vi "1D experiment wii.vi"() -> ()   [LabVIEW 2011]
uses:
  <vilib>/Platform/TimedLoop/XDataNode/timing_clust.ctl
  <vilib>/Platform/TimedLoop/XDataNode/nitl_modes.ctl
  <vilib>/Platform/TimedLoop/XDataNode/wakeup.ctl
  3D_Experiment/libs/experiments 2/Action Engines/AE Access VIs/AE - Bluetooth Initialise.vi
  3D_Experiment/libs/experiments 2/Action Engines/AE Access VIs/AE - Bluetooth Connect All.vi
  <vilib>/Utility/inputDevices.llb/closeMouse.vi
  <vilib>/Utility/cursorutil.llb/Set Cursor (Cursor ID).vi
  <vilib>/Utility/inputDevices.llb/mouseAcquire.vi
  <vilib>/Utility/file.llb/Write To Spreadsheet File (DBL).vi
  <vilib>/Utility/file.llb/Write To Spreadsheet File (I64).vi
  <vilib>/Platform/TimedLoop/XDataNode/XDataNode.xnode
  <vilib>/Platform/TimedLoop/XDataNode/XDNodeRunTimeDep.lvlib
  User32.dll
panel:
  out "initial time":u32
  out "1D Experiment":cluster{"Y":dbl[], "Y":dbl[]}[](graph)
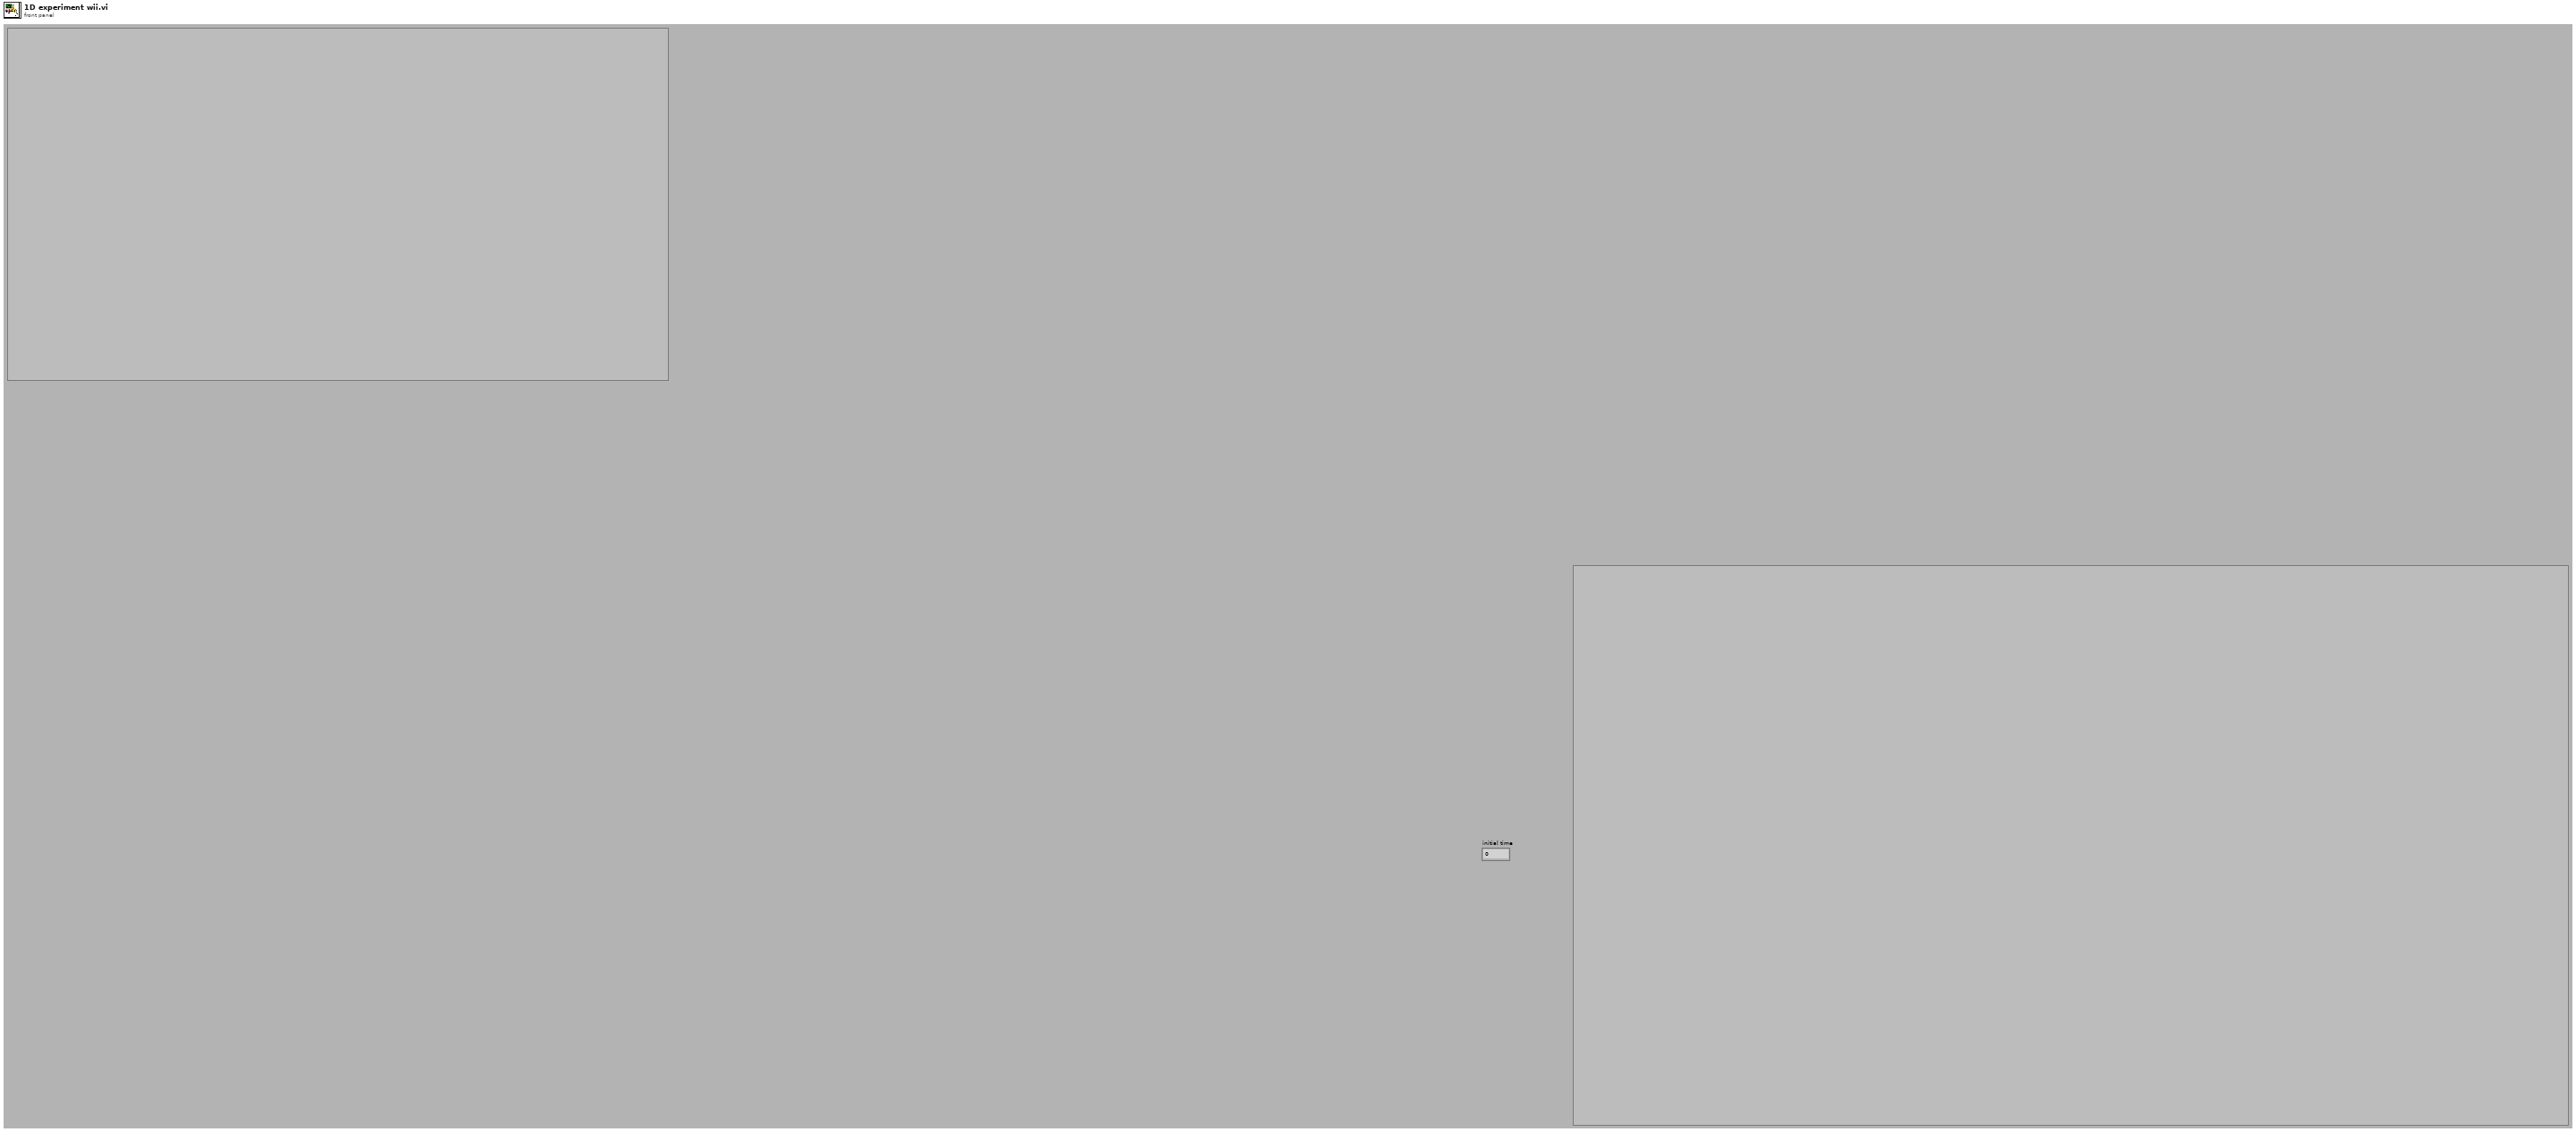
[diagram p1: front panel]
types:
  T1 = enum16{"open", "replace", "create", "open or create", "replace or create", "replace or create with confirmation"}
  T2 = typedef "XDNodeRunTimeDep.lvlib/timing_clust.ctl" = cluster{"Expected End [f-1]":u64, "Actual End [f-1]":u64, "Finished Late? [f-1]":bool, "Expected End [i-1]":u64, "Actual End [i-1]":u64, "Finished Late? [i-1]":bool, "Expected Start [i]":u64, "Actual Start [i]":u64, "Expected Start [f]":u64, "Actual Start [f]":u64, "Source Name":string, "Structure Name":string, "Period":i64, "Deadline":i64, "Offset":i64, "Start":i64, "Priority":i32, "Timeout":i32, "Mode":T3, "Wakeup Reason":T4, "Error":errorcluster, "Source Type":string, "Secondary Source Type":string, "Global End Time":u64, "Global Start Time":u64, "Frame Duration":u64, "Iteration Duration":u64, "Assigned CPU":i32, "I/O Scan Engine Mode":u32}
  T3 = typedef "XDNodeRunTimeDep.lvlib/nitl_modes.ctl" = enum32{"No Change", "Process missed periods, maintain original phase", "Discard missed periods, maintain original phase", "Process missed periods, ignore original phase", "Discard missed periods, ignore original phase"}
  T4 = typedef "XDNodeRunTimeDep.lvlib/wakeup.ctl" = enum32{"Normal", "Aborted", "Asynchronous wakeup", "Timing source error", "Timed loop error", "Timeout"}
  T5 = cluster{"Radius":dbl, "x0":dbl, "y0":dbl, "D":dbl, bool}
  T6 = typedef "LVAllMonitorsDisplayTypeDef.ctl" = cluster{"Bounds":cluster{"Left":i16, "Top":i16, "Right":i16, "Bottom":i16}, "Depth":i16}[]
  T7 = cluster{"Bounds":cluster{"Left":i16, "Top":i16, "Right":i16, "Bottom":i16}, "Depth":i16}
  T8 = cluster{"Left":i16, "Top":i16, "Right":i16, "Bottom":i16}
  T9 = cluster{"Horizontal":i32, "Vertical":i32, "Scrolling":i32}
  T10 = cluster{"button 1":bool, "button 2":bool, "button 3":bool, "button 4":bool}
  T11 = typedef "LVPoint32TypeDef.ctl" = cluster{"Horizontal":i32, "Vertical":i32}
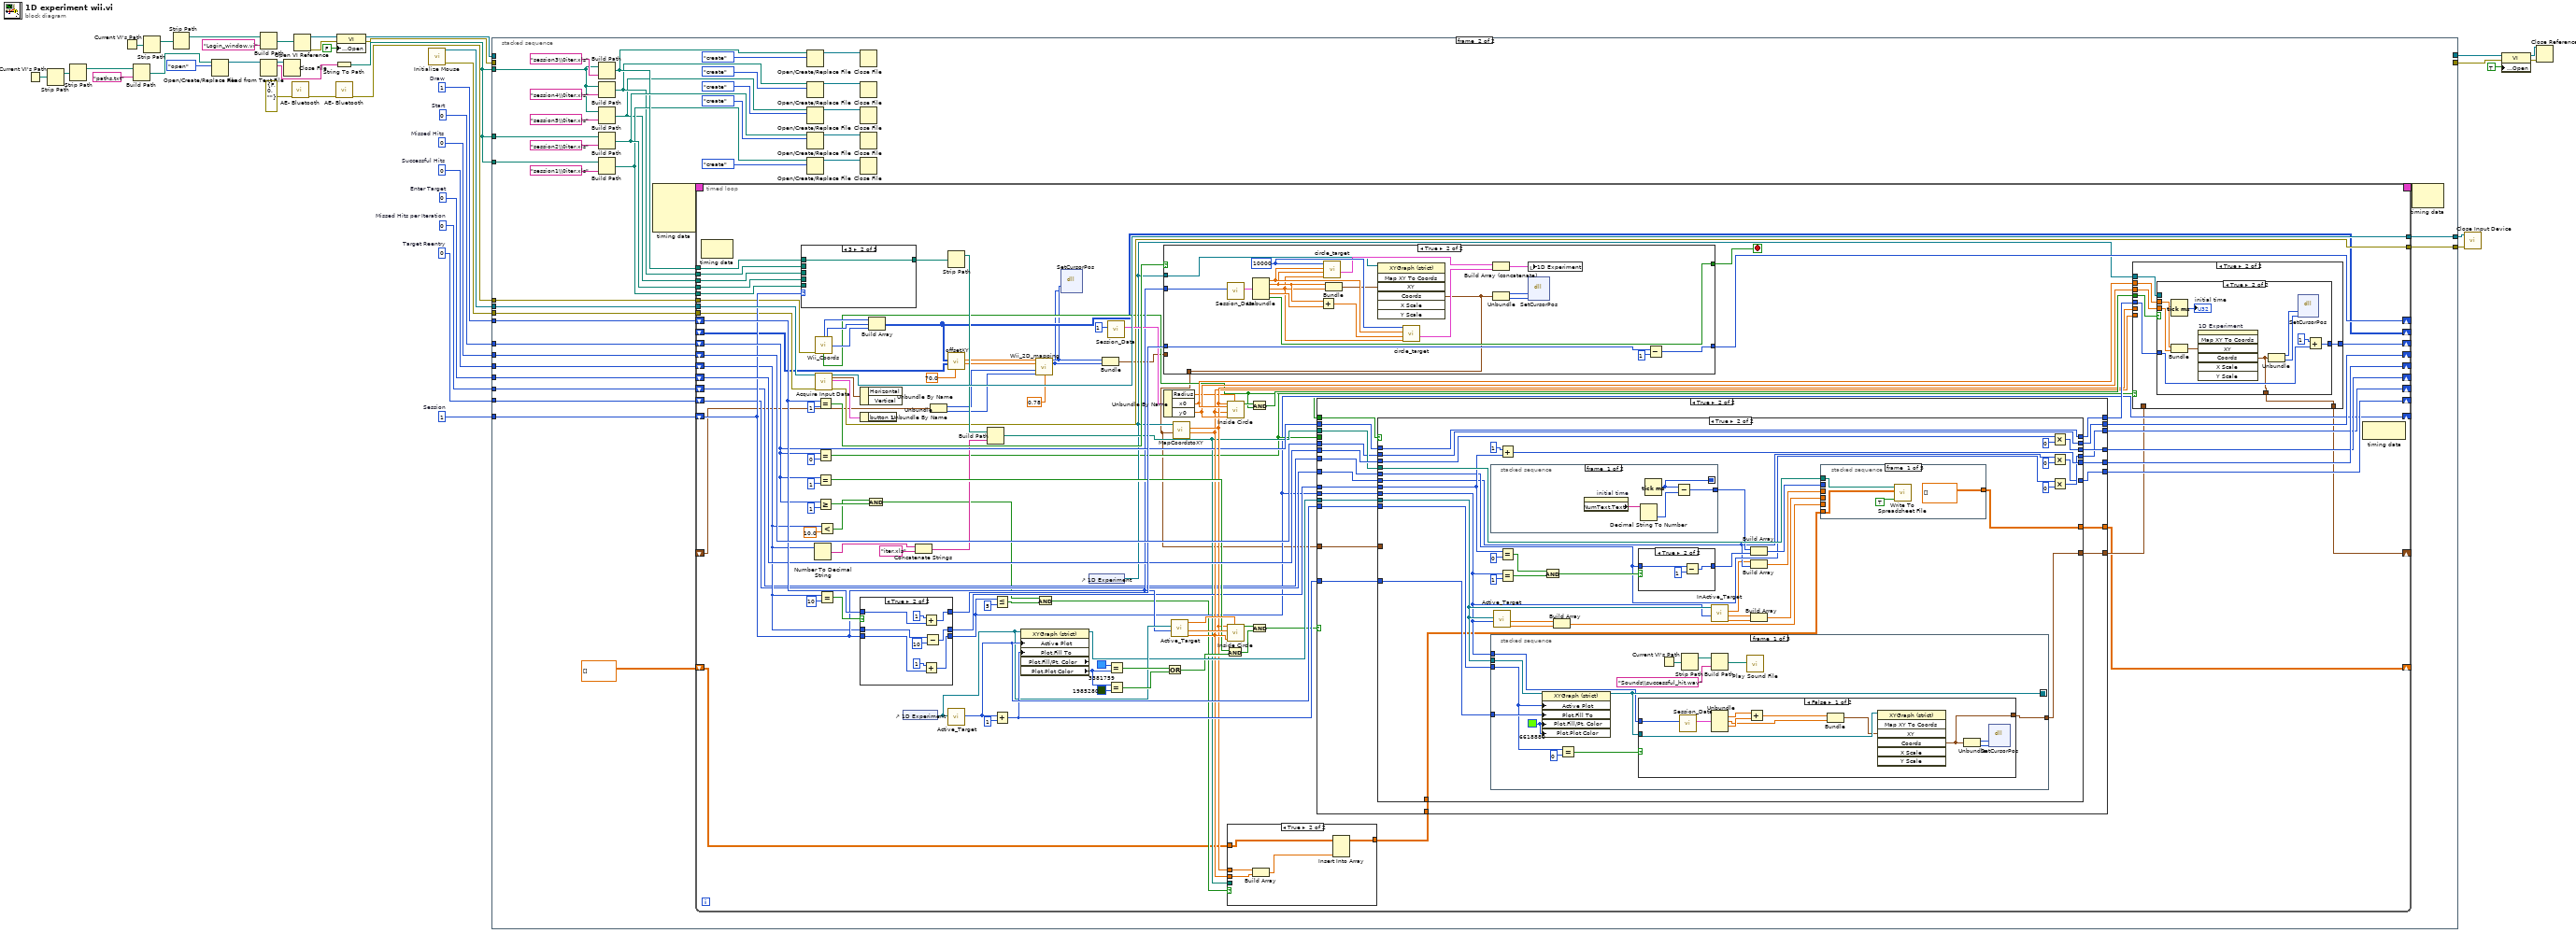
[diagram p0: block diagram]
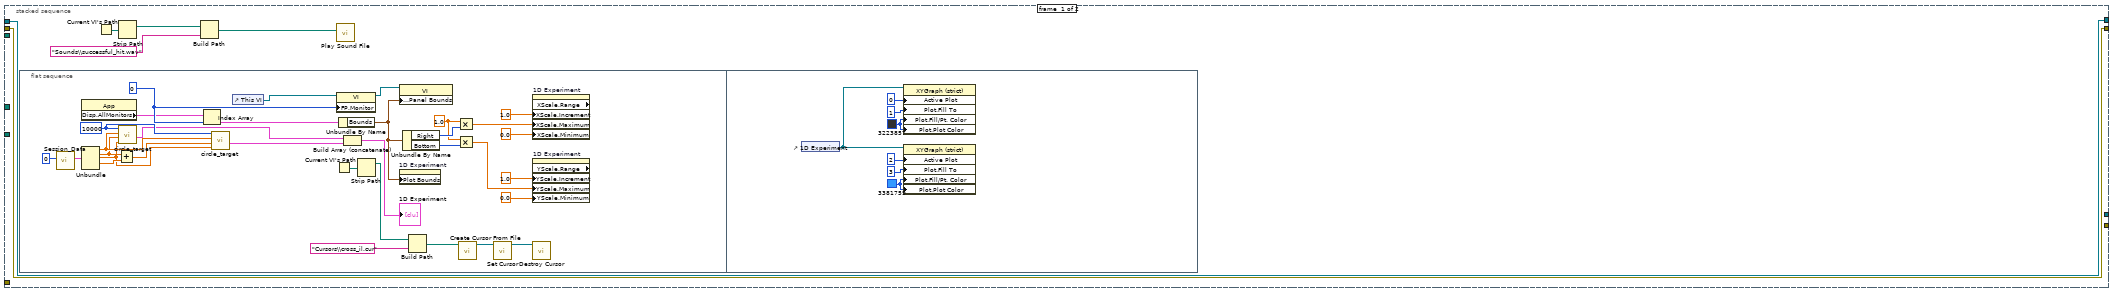
[diagram p2: hidden frame]
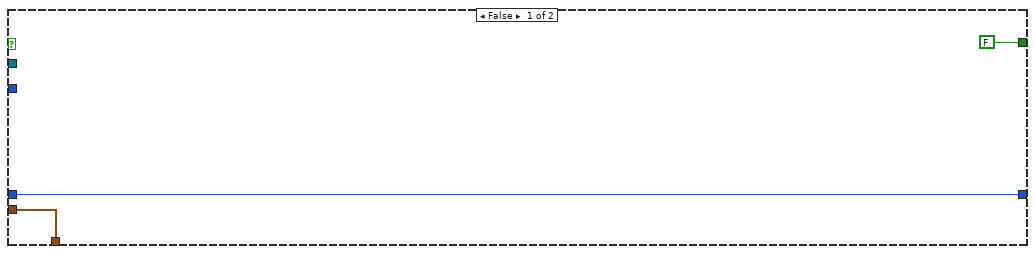
[diagram p8: hidden frame]
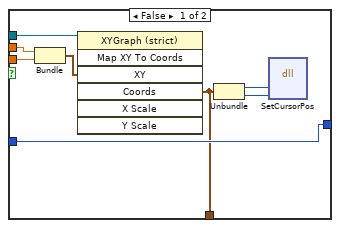
[diagram p10: hidden frame]
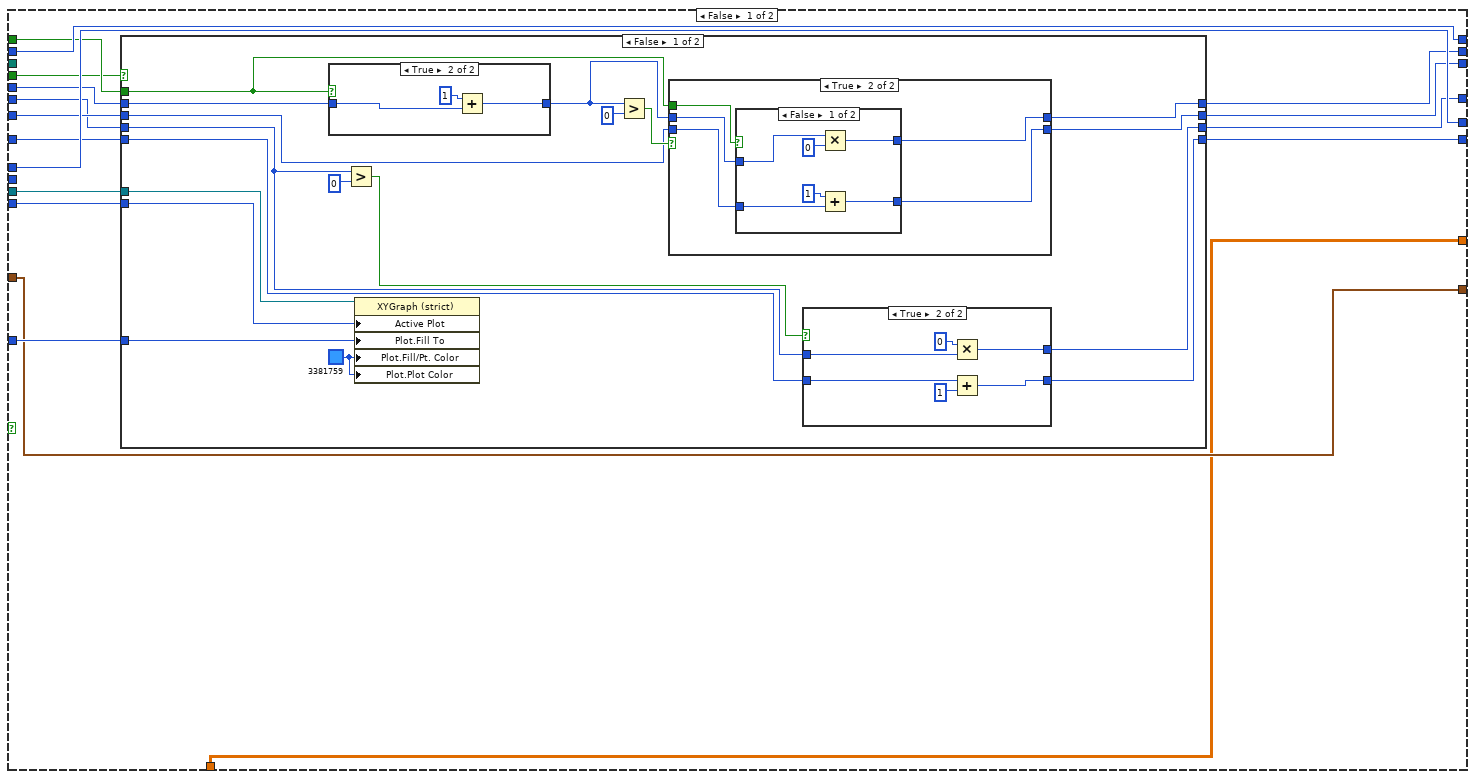
[diagram p12: hidden frame]
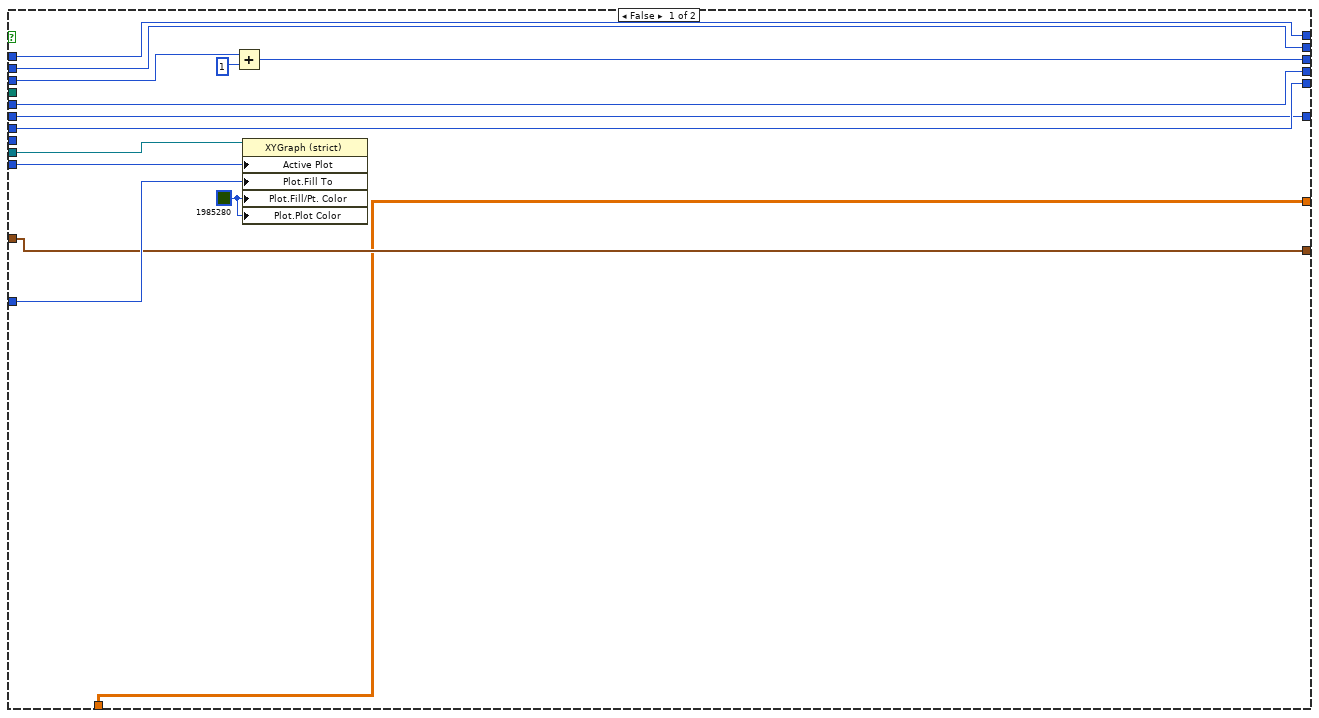
[diagram p18: hidden frame]
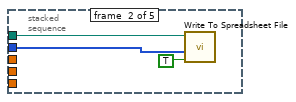
[diagram p20: hidden frame]
diagram:
  w6 = 0  # Target Reentry
  w7 = 0  # Missed Hits per Iteration
  w33 = 0  # Enter Target
  w34 = 1  # Draw
  w35 = 0  # Start
  w36 = 1  # Session
  w37 = 0  # Missed Hits
  w38 = 0  # Successful Hits
  n1 = Current VI's Path() -> (path=w15:path)
  n2 = Strip Path(path=w15) -> (stripped path=w10:path)  [unwired: 1 out]
  n3 = Strip Path(path=w10) -> (stripped path=w11:path)  [unwired: 1 out]
  n4 = Current VI's Path() -> (path=w18:path)
  n5 = Build Path(base path=w11, name or relative path="paths.txt") -> (appended path=w13:path)
  n6 = Strip Path(path=w18) -> (stripped path=w8:path)  [unwired: 1 out]
  n7 = Strip Path(path=w8) -> (stripped path=w9:path)  [unwired: 1 out]
  n8 = Open/Create/Replace File(file path (use dialog)=w13, operation (0:open)=T1."open") -> (refnum out=w31:refnum<file>)  [unwired: 4 in, 2 out]
  n9 = Build Path(base path=w9, name or relative path="Login_window.vi") -> (appended path=w16:path)
  n10 = Read from Text File(file (use dialog)=w31) -> (refnum out=w32:refnum<file>, text=w30:string)  [unwired: 3 in, 2 out]
  n11 = Close File(refnum=w32) -> ()  [unwired: 1 in, 2 out]
  n12 = call-poly "AE- Bluetooth.vi"("error in (no error)"=errorcluster {"status"=FALSE, "code"=0, "source"=""}) -> ("error out"=w2:errorcluster)  [unwired: 10 in]
  n13 = Open VI Reference(vi path=w16) -> (vi reference=w28:refnum<vi>, error out=w27:errorcluster)  [unwired: 5 in]
  n14 = String To Path(string=w30) -> (path=w29:path)
  n15 = call-poly "AE- Bluetooth.vi"("error in (no error)"=w2) -> ("error out"=w1:errorcluster)  [unwired: 9 in, 1 out]
  n16 = property class="VI"(reference=w28, error in=w27, "Front Panel Window:Open"=FALSE) -> (reference out=w25:refnum<vi>, error out=w24:errorcluster)
  n17 = call <vilib>:"Initialize Mouse.vi"() -> ("error out"=w5:errorcluster, "device ID"=w40:refnum<k1>)  [unwired: 1 in, 9 out]
  n18 = stacked-sequence {
    tunnel: w40 -> [_ w124]
    tunnel: [_ w123] -> w39
    tunnel: w38 -> [_ w122]
    tunnel: w37 -> [_ w121]
    tunnel: w36 -> [_ w117]
    tunnel: w35 -> [_ w120]
    tunnel: w34 -> [_ w119]
    tunnel: w33 -> [_ w118]
    tunnel: w29 -> [_ w107]
    tunnel: w29 -> [_ w114]
    tunnel: w29 -> [_ w94]
    tunnel: w25 -> [w42 _]
    tunnel: w24 -> [w41 _]
    tunnel: [w42 _] -> w20
    tunnel: [w41 _] -> w19
    tunnel: w7 -> [_ w100]
    tunnel: w6 -> [_ w99]
    tunnel: w5 -> [_ w98]
    tunnel: [_ w97] -> w4
    tunnel: w1 -> [_ w87]
    frame #0 {
      n19 = flat-sequence {
        frame #0 {
          w64 = 1.0 ("y")
          w69 = u16 0 ("Front Panel Window:Monitor")
          w78 = 10000
          n20 = call "Session_Data.vi"("Session"=0) -> ("output cluster"=w56:T5)  [unwired: 10 in]
          n21 = property class="App"() -> ("Disp.AllMonitors"=w68:T6)  [unwired: 2 in, 2 out]
          n22 = Unbundle(w56) -> ("Radius"=w76:dbl, "x0"=w54:dbl, "y0"=w53:dbl, "D"=w55:dbl)  [unwired: 1 out]
          n23 = Add(x=w54, y=w55) -> (x+y=w77:dbl)
          n24 = call "circle_target.vi"("y0"=w53, "x0"=w54, "Radius"=w76, "Pixels"=w78) -> ("Target plots"=w74:cluster{dbl[], dbl[]}[])  [unwired: 7 in]
          n25 = Index Array(array=w68, index=w69) -> (element=w70:T7)
          n26 = call "circle_target.vi"("y0"=w53, "x0"=w77, "Radius"=w76, "Pixels"=w78) -> ("Target plots"=w75:cluster{dbl[], dbl[]}[])  [unwired: 7 in]
          n27 = control-ref of="This VI"() -> (w71:refnum<vi>)
          n28 = Current VI's Path() -> (path=w52:path)
          n29 = property class="VI"(reference=w71, "FP.Monitor"=w69) -> (reference out=w67:refnum<vi>)  [unwired: 1 in, 1 out]
          n30 = Unbundle By Name(w70) -> ("Bounds"=w66:T8)
          n31 = Build Array (concatenate)(w74, w75) -> (→"1D Experiment":cluster{dbl[], dbl[]}[])
          n32 = Strip Path(path=w52) -> (stripped path=w51:path)  [unwired: 1 out]
          n33 = property class="VI"(reference=w67, "Front Panel Window:Panel Bounds"=w66) -> ()  [unwired: 1 in, 2 out]
          n34 = property on="1D Experiment" class="XYGraph (strict)"("Plot Bounds"=w66) -> ()  [unwired: 2 in, 2 out]
          n35 = Unbundle By Name(w66) -> ("Right"=w65:i16, "Bottom"=w63:i16)
          n36 = Build Path(base path=w51, name or relative path="Cursors\\cross_il.cur") -> (appended path=w49:path)
          n37 = Multiply(x=w64, y=w65) -> (x*y=w61:dbl)
          n38 = Multiply(x=w64, y=w63) -> (x*y=w58:dbl)
          n39 = call <vilib>:"Create Cursor From File.vi"("cursor file"=w49) -> ("cursor ID"=w48:refnum<k1>)  [unwired: 9 in, 1 out]
          n40 = call-poly <vilib>:"Set Cursor.vi"("cursor ID"=w48) -> ("previous cursor ID"=w47:refnum<k1>)  [unwired: 9 in, 1 out]
          n41 = property on="1D Experiment" class="XYGraph (strict)" props=["XScale", "Range", "XScale", "Increment", "XScale", "Maximum", "XScale", "Minimum"]("XScale.Increment"=1.0 ("X Scale.Range:Increment"), "XScale.Maximum"=w61, "XScale.Minimum"=0.0 ("X Scale.Range:Minimum")) -> ()  [unwired: 2 in, 3 out]
          n42 = property on="1D Experiment" class="XYGraph (strict)" props=["YScale", "Range", "YScale", "Increment", "YScale", "Maximum", "YScale", "Minimum"]("YScale.Increment"=1.0 ("Y Scale.Range:Increment"), "YScale.Maximum"=w58, "YScale.Minimum"=0.0 ("Y Scale.Range:Minimum")) -> ()  [unwired: 2 in, 3 out]
          n43 = call <vilib>:"Destroy Cursor.vi"("cursor ID"=w47) -> ()  [unwired: 9 in, 1 out]
        }
        frame #1 {
          w84 = u32 3381759
          w81 = u32 3223857
          n44 = control-ref of="1D Experiment"() -> (w85:refnum<vi>)
          n45 = property on="Property Node" class="XYGraph (strict)"(reference=w85, "Active Plot"=u32 0, "Plot.Fill To"=i16 1, "Plot.Fill/Pt. Color"=w81, "Plot.Plot Color"=w81) -> ()  [unwired: 1 in, 2 out]
          n46 = property on="Property Node" class="XYGraph (strict)"(reference=w85, "Active Plot"=u32 2, "Plot.Fill To"=i16 3, "Plot.Fill/Pt. Color"=w84, "Plot.Plot Color"=w84) -> ()  [unwired: 1 in, 2 out]
        }
      }
      n47 = Current VI's Path() -> (path=w44:path)
      n48 = Strip Path(path=w44) -> (stripped path=w43:path)  [unwired: 1 out]
      n49 = Build Path(base path=w43, name or relative path="Sounds\\successful_hit.wav") -> (appended path=w45:path)
      n50 = call <vilib>:"Play Sound File.vi"("path"=w45) -> ()  [unwired: 9 in, 2 out]
    }
    frame #1 {
      n51 = Build Path(base path=w94, name or relative path="session3\\0iter.xls") -> (appended path=w108:path)
      n52 = Build Path(base path=w94, name or relative path="session4\\0iter.xls") -> (appended path=w89:path)
      n53 = Build Path(base path=w94, name or relative path="session5\\0iter.xls") -> (appended path=w88:path)
      n54 = Build Path(base path=w114, name or relative path="session2\\0iter.xls") -> (appended path=w111:path)
      n55 = Build Path(base path=w107, name or relative path="session1\\0iter.xls") -> (appended path=w103:path)
      n56 = node-c288() -> (w102:T2)  [unwired: 4 in]
      n57 = timed-loop {
        tunnel: w124 -> [w217]
        tunnel: [w216] -> w123
        shift-right: [w214] -> _
        shift-left: w122 -> [w165]
        shift-right: [w212] -> _
        shift-left: w121 -> [w213]
        shift-right: [w156] -> _
        shift-left: w117 -> [w178]
        shift-right: [w204] -> _
        shift-left: w120 -> [w181]
        shift-right: [w198] -> _
        shift-left: w119 -> [w199]
        shift-right: [w194] -> _
        shift-left: w118 -> [w195]
        tunnel: w103 -> [w179]
        tunnel: w111 -> [w177]
        tunnel: w108 -> [w176]
        timing: w102 -> [_]
        timing-out: [_] -> w101
        shift-right: [w161] -> _
        shift-left: w100 -> [w163]
        shift-right: [w159] -> _
        shift-left: w99 -> [w160]
        tunnel: w98 -> [w151]
        tunnel: [w150] -> w97
        tunnel: w89 -> [w149]
        tunnel: w88 -> [w148]
        tunnel: w87 -> [w143]
        shift-right: [w139] -> _
        shift-left: _ -> [w138]
        shift-right: [w130] -> _
        shift-left: _ -> [w134]
        shift-right: [w125] -> _
        shift-left: dbl[][] [] -> [w127]
        stop <- w188 stop-if-true
        n58 = node-c288() -> ()  [unwired: 1 in, 1 out]
        n59 = case shown="3" w178 {
          tunnel: w179 -> [_ _ _ _ w234]
          tunnel: [w230 w231 w232 w233 w234] -> w174
          tunnel: w177 -> [w230 _ _ _ _]
          tunnel: w176 -> [_ w231 _ _ _]
          tunnel: w149 -> [_ _ w232 _ _]
          tunnel: w148 -> [_ _ _ w233 _]
          frame 2 {
          }
          frame 3 {
          }
          frame 4 {
          }
          frame 5 {
          }
          frame 1, Default {
          }
        }
        n60 = Number To Decimal String(number=w165) -> (decimal integer string=w173:string)  [unwired: 1 in]
        n61 = call "Wii_Coords.vi"("error in (no error)"=w143) -> ("Raw X Values"=w147:i32[], "Raw Y Values"=w146:i32[], "Sizes"=w145:i32[], "B"=w142:bool)  [unwired: 7 in, 4 out]
        n62 = call-poly <vilib>:"Acquire Input Data.vi"("device ID"=w217, "error in (no error)"=w151) -> ("device ID"=w216:refnum<k1>, "axis info"=w215:T9, "button info"=w218:T10, "error out"=w150:errorcluster)  [unwired: 1 in, 13 out]
        n63 = Equal?(x=w199, y=1) -> (x = y?=w196:bool)
        n64 = Equal?(x=w181, y=0) -> (x = y?=w162:bool)
        n65 = Equal?(x=w181, y=1) -> (x = y?=w190:bool)
        n66 = Greater Or Equal?(x=w181, y=1) -> (x >= y?=w168:bool)
        n67 = Less?(x=w165, y=10.0) -> (x < y?=w167:bool)
        n68 = Equal?(x=w165, y=10) -> (x = y?=w210:bool)
        n69 = Unbundle By Name(w215) -> ()  [unwired: 2 out]
        n70 = Unbundle By Name(w218) -> ()  [unwired: 1 out]
        n71 = case shown="True" w210 {
          tunnel: w165 -> [w293 w302]
          tunnel: [w293 w300] -> w175
          tunnel: w178 -> [w292 w294]
          tunnel: [w292 w295] -> w156
          tunnel: w199 -> [w291 w298]
          tunnel: [w291 w296] -> w197
          frame False {
          }
          frame True {
            n72 = Add(x=1, y=w298) -> (x+y=w296:i32)
            n73 = Add(x=1, y=w294) -> (x+y=w295:i32)
            n74 = Subtract(x=w302, y=10) -> (x-y=w300:i32)
          }
        }
        n75 = And(x=w167, y=w168) -> (x .and. y?=w157:bool)
        n76 = Build Array(w147, w146, w145) -> (w139:i32[][])
        n77 = control-ref of="1D Experiment"() -> (w208:refnum<vi>)
        n78 = Concatenate Strings(w173, "iter.xls" ("name or relative path")) -> (w171:string)
        n79 = Unbundle(w134) -> ("Horizontal"=w133:i32, "Vertical"=w132:i32)
        n80 = Strip Path(path=w174) -> (stripped path=w170:path)  [unwired: 1 out]
        n81 = call "offsetXY.vi"("Thres"=70.0, "Previous"=w138, "Current"=w139) -> ("OffsetY"=w141:dbl, "OffsetX"=w140:dbl)  [unwired: 7 in]
        n82 = call "Active_Target.vi"("XYGraph Refnum"=w208) -> ("Active Plot"=w222:u32)  [unwired: 7 in, 3 out]
        n83 = Build Path(base path=w170, name or relative path=w171) -> (appended path=w169:path)
        n84 = Less Or Equal?(x=w156, y=5) -> (x <= y?=w153:bool)
        n85 = Add(x=w222, y=u32 1) -> (x+y=w221:u32)
        n86 = property on="Property Node" class="XYGraph (strict)" props=["Active Plot", "Plot", "Fill To", "Plot", "Fill/Pt. Color", "Plot", "Plot Color"](reference=w208, "Active Plot"=w222, "Plot.Fill To"=w221) -> (reference out=w201:refnum<vi>, "Plot.Plot Color"=w203:u32)  [unwired: 1 in, 2 out]
        n87 = call "Wii_2D_mapping.vi"("Wii_X_off"=w140, "Wii_Y_off"=w141, "previous_X"=w133, "previous_Y"=w132, "X_Y_speed"=0.78) -> ("X"=w136:i32, "Y"=w135:i32)  [unwired: 9 in]
        n88 = And(x=w157, y=w153) -> (x .and. y?=w154:bool)
        n89 = dll-call lib="User32.dll" fn="SetCursorPos"(w136, w135) -> ()  [unwired: 6 in, 2 out]
        n90 = control-ref of="1D Experiment"() -> (w164:refnum<vi>)
        n91 = Bundle("X"=w136, "Y"=w135) -> (w129:cluster{"X":i32, "Y":i32})  [unwired: 1 in]
        n92 = call "Session_Data.vi"("Session"=1) -> ("output cluster"=w187:T5)  [unwired: 10 in]
        n93 = Equal?(x=u32 3381759, y=w203) -> (x = y?=w225:bool)
        n94 = Equal?(x=w203, y=u32 1985280) -> (x = y?=w224:bool)
        n95 = case shown="True" w196 {
          tunnel: w178 -> [_ w252]
          tunnel: [w242 w262] -> w198
          tunnel: w197 -> [w242 w261]
          tunnel: [FALSE ("Valid") w251] -> w188
          tunnel: w164 -> [_ w248]
          tunnel: w129 -> [w241 _]
          tunnel: [w241 w244] -> w128
          frame False {
          }
          frame True {
            w260 = 10000
            n96 = call "Session_Data.vi"("Session"=w252) -> ("output cluster"=w255:T5)  [unwired: 10 in]
            n97 = Unbundle(w255) -> ("Radius"=w258:dbl, "x0"=w247:dbl, "y0"=w246:dbl, "D"=w254:dbl, w251:bool)
            n98 = Add(x=w247, y=w254) -> (x+y=w259:dbl)
            n99 = call "circle_target.vi"("y0"=w246, "x0"=w247, "Radius"=w258, "Pixels"=w260) -> ("Target plots"=w256:cluster{dbl[], dbl[]}[])  [unwired: 7 in]
            n100 = Bundle("x0"=w247, "y0"=w246) -> (w245:cluster{"x0":dbl, "y0":dbl})  [unwired: 1 in]
            n101 = invoke on="Invoke Node" class="XYGraph (strict)" method="Map XY To Coords"(reference=w248, "XY"=w245) -> ("Coords"=w244:T11)  [unwired: 5 in, 6 out]
            n102 = call "circle_target.vi"("y0"=w246, "x0"=w259, "Radius"=w258, "Pixels"=w260) -> ("Target plots"=w257:cluster{dbl[], dbl[]}[])  [unwired: 7 in]
            n103 = Build Array (concatenate)(w256, w257) -> (w253:cluster{dbl[], dbl[]}[])
            n104 = Unbundle(w244) -> ("Horizontal"=w250:i32, "Vertical"=w249:i32)
            n105 = local write "1D Experiment"(w253) -> ()
            n106 = dll-call lib="User32.dll" fn="SetCursorPos"(w250, w249) -> ()  [unwired: 6 in, 2 out]
            n107 = Subtract(x=w261, y=1) -> (x-y=w262:i32)
          }
        }
        n108 = Unbundle By Name(w187) -> ("Radius"=w158:dbl, "x0"=w186:dbl, "y0"=w185:dbl)
        n109 = Or(x=w225, y=w224) -> (x .or. y?=w192:bool)
        n110 = call "Active_Target.vi"("Session"=w178, "XYGraph Refnum"=w208) -> ("y0"=w219:dbl, "x0"=w220:dbl, "Radius"=w209:dbl)  [unwired: 6 in, 1 out]
        n111 = call "MapCoordstoXY.vi"("Coordinates"=w128, "XYGraph Refnum"=w164) -> ("Y(graph)"=w182:dbl, "X (graph)"=w183:dbl)  [unwired: 7 in]
        n112 = And(x=w190, y=w192) -> (x .and. y?=w189:bool)
        n113 = call "Inside Circle.vi"("Radius"=w158, "y0"=w185, "y"=w182, "x0"=w186, "x"=w183) -> ("Inside Circle"=w206:bool)  [unwired: 6 in]
        n114 = call "Inside Circle.vi"("Radius"=w209, "y0"=w219, "y"=w182, "x0"=w220, "x"=w183) -> ("Inside Circle"=w191:bool)  [unwired: 6 in]
        n115 = case shown="True" w154 {
          tunnel: w183 -> [_ w240]
          tunnel: w182 -> [_ w239]
          tunnel: w169 -> [_ _]
          tunnel: w127 -> [w235 w237]
          tunnel: [w235 w236] -> w126
          frame False {
          }
          frame True {
            n116 = Build Array(w240, w239) -> (w238:dbl[])
            n117 = Insert Into Array(array=w237, new element=w238) -> (w236:dbl[][])  [unwired: 2 in]
          }
        }
        n118 = And(x=w206, y=w142) -> (x .and. y?=w205:bool)
        n119 = And(x=w191, y=w189) -> (x .and. y?=w152:bool)
        n120 = case shown="True" w152 {
          tunnel: w142 -> [w313 w390]
          tunnel: w222 -> [w317 w387]
          tunnel: w221 -> [w316 w386]
          tunnel: w175 -> [w319 w389]
          tunnel: [w319 w388] -> w214
          tunnel: w213 -> [w318 w378]
          tunnel: [w310 w376] -> w212
          tunnel: w181 -> [w315 w385]
          tunnel: [w315 w384] -> w202
          tunnel: w201 -> [w314 w383]
          tunnel: w195 -> [w308 w382]
          tunnel: [w307 w381] -> w194
          tunnel: w156 -> [_ w380]
          tunnel: w169 -> [_ w379]
          tunnel: w163 -> [w312 w377]
          tunnel: w162 -> [w311 _]
          tunnel: [w309 w375] -> w161
          tunnel: w160 -> [w306 w374]
          tunnel: [w305 w373] -> w159
          tunnel: w128 -> [w304 w372]
          tunnel: [w304 w371] -> w131
          tunnel: w126 -> [w303 w370]
          tunnel: [w303 w369] -> w125
          frame False {
            n121 = case shown="False" w311 {
              tunnel: w318 -> [w336 w367]
              tunnel: w317 -> [w335 _]
              tunnel: w316 -> [w334 _]
              tunnel: w314 -> [w333 _]
              tunnel: w313 -> [w330 _]
              tunnel: w312 -> [w328 w368]
              tunnel: [w327 w367] -> w310
              tunnel: [w326 w368] -> w309
              tunnel: w308 -> [w323 w366]
              tunnel: [w322 w366] -> w307
              tunnel: w306 -> [w321 w365]
              tunnel: [w320 w365] -> w305
              frame False {
                w337 = u32 3381759
                n122 = case shown="True" w330 {
                  tunnel: w336 -> [w361 w364]
                  tunnel: [w361 w362] -> w329
                  frame False {
                  }
                  frame True {
                    n123 = Add(x=1, y=w364) -> (x+y=w362:i32)
                  }
                }
                n124 = Greater?(x=w323, y=0) -> (0:w324:bool)
                n125 = property on="Property Node" class="XYGraph (strict)"(reference=w333, "Active Plot"=w335, "Plot.Fill To"=w334, "Plot.Fill/Pt. Color"=w337, "Plot.Plot Color"=w337) -> ()  [unwired: 1 in, 2 out]
                n126 = Greater?(x=w329, y=0) -> (0:w331:bool)
                n127 = case shown="True" w331 {
                  tunnel: [w346 w352] -> w326
                  tunnel: [w347 w351] -> w327
                  tunnel: w330 -> [_ w350]
                  tunnel: w329 -> [w347 w349]
                  tunnel: w328 -> [w346 w348]
                  frame False {
                  }
                  frame True {
                    n128 = case shown="False" w350 {
                      tunnel: [w357 w360] -> w352
                      tunnel: [w355 w359] -> w351
                      tunnel: w349 -> [w354 w359]
                      tunnel: w348 -> [w353 w360]
                      frame False {
                        n129 = Multiply(x=w354, y=0) -> (x*y=w355:i32)
                        n130 = Add(x=1, y=w353) -> (x+y=w357:i32)
                      }
                      frame True {
                      }
                    }
                  }
                }
                n131 = case shown="True" w324 {
                  tunnel: w323 -> [w339 w345]
                  tunnel: [w339 w343] -> w322
                  tunnel: w321 -> [w338 w342]
                  tunnel: [w338 w340] -> w320
                  frame False {
                  }
                  frame True {
                    n132 = Multiply(x=0, y=w345) -> (x*y=w343:i32)
                    n133 = Add(x=w342, y=1) -> (x+y=w340:i32)
                  }
                }
              }
              frame True {
              }
            }
          }
          frame True {
            n134 = case shown="True" w390 {
              tunnel: w389 -> [w403 w418]
              tunnel: [w403 w438] -> w388
              tunnel: w387 -> [w402 w441]
              tunnel: w386 -> [w401 w440]
              tunnel: w385 -> [w399 w439]
              tunnel: [w399 w439] -> w384
              tunnel: w383 -> [w400 w425]
              tunnel: w382 -> [w395 w430]
              tunnel: [w396 w428] -> w381
              tunnel: w380 -> [_ w416]
              tunnel: w379 -> [_ w436]
              tunnel: w378 -> [w398 w434]
              tunnel: [w398 w434] -> w376
              tunnel: w377 -> [w397 w411]
              tunnel: [w397 w432] -> w375
              tunnel: w374 -> [w393 w409]
              tunnel: [w393 w427] -> w373
              tunnel: [w392 w407] -> w371
              tunnel: w372 -> [w392 _]
              tunnel: w370 -> [w391 w406]
              tunnel: [w391 w405] -> w369
              frame False {
                w404 = u32 1985280
                n135 = Add(x=w395, y=1) -> (x+y=w396:i32)
                n136 = property on="Property Node" class="XYGraph (strict)"(reference=w400, "Active Plot"=w402, "Plot.Fill To"=w401, "Plot.Fill/Pt. Color"=w404, "Plot.Plot Color"=w404) -> ()  [unwired: 1 in, 2 out]
              }
              frame True {
                n137 = stacked-sequence {
                  seq-local: [w463 _] -> [_ w467]
                  tunnel: [w464 _] -> w435
                  frame #0 {
                    n138 = property on="initial time" class="DigNum (strict)"() -> ("NumText.Text"=w466:string)  [unwired: 2 in, 2 out]
                    n139 = Decimal String To Number(string=w466) -> (number=w465:i32)  [unwired: 2 in, 1 out]
                    n140 = Tick Count (ms)() -> (millisecond timer value=w463:u32)
                    n141 = Subtract(x=w463, y=w465) -> (x-y=w464:u32)
                  }
                  frame #1 {
                    n142 = Number To Decimal String(number=w467) -> (decimal integer string=w468:string)  [unwired: 1 in]
                    n143 = property on="initial time" class="DigNum (strict)"("NumText.Text"=w468) -> ()  [unwired: 2 in, 2 out]
                  }
                }
                n144 = stacked-sequence {
                  seq-local: [w478 _ _] -> [_ w502 w511]
                  tunnel: w441 -> [w477 w503 w513]
                  tunnel: w440 -> [w480 _ w512]
                  tunnel: w425 -> [w479 _ _]
                  tunnel: w416 -> [w474 _ _]
                  tunnel: [w469 _ _] -> w407
                  frame #0 {
                    w481 = u32 6618880
                    n145 = property on="Property Node" class="XYGraph (strict)"(reference=w479, "Active Plot"=w477, "Plot.Fill To"=w480, "Plot.Fill/Pt. Color"=w481, "Plot.Plot Color"=w481) -> (reference out=w478:refnum<vi>)  [unwired: 1 in, 1 out]
                    n146 = Equal?(x=w477, y=u32 0) -> (x = y?=w475:bool)
                    n147 = case shown="False" w475 {
                      tunnel: w478 -> [w489 w495]
                      tunnel: w474 -> [w487 w499]
                      tunnel: [w482 w493] -> w469
                      frame False {
                        n148 = call "Session_Data.vi"("Session"=w487) -> ("output cluster"=w490:T5)  [unwired: 10 in]
                        n149 = Unbundle(w490) -> ("x0"=w485:dbl, "y0"=w483:dbl, "D"=w484:dbl)  [unwired: 2 out]
                        n150 = Add(x=w485, y=w484) -> (x+y=w486:dbl)
                        n151 = Bundle(w486, "y0"=w483) -> (w488:cluster{dbl, "y0":dbl})  [unwired: 1 in]
                        n152 = invoke on="Invoke Node" class="XYGraph (strict)" method="Map XY To Coords"(reference=w489, "XY"=w488) -> ("Coords"=w482:T11)  [unwired: 5 in, 6 out]
                        n153 = Unbundle(w482) -> ("Horizontal"=w492:i32, "Vertical"=w491:i32)
                        n154 = dll-call lib="User32.dll" fn="SetCursorPos"(w492, w491) -> ()  [unwired: 6 in, 2 out]
                      }
                      frame True {
                        n155 = call "Session_Data.vi"("Session"=w499) -> ("output cluster"=w498:T5)  [unwired: 10 in]
                        n156 = Unbundle(w498) -> ("x0"=w497:dbl, "y0"=w494:dbl)  [unwired: 3 out]
                        n157 = Bundle("x0"=w497, "y0"=w494) -> (w496:cluster{"x0":dbl, "y0":dbl})  [unwired: 1 in]
                        n158 = invoke on="Invoke Node" class="XYGraph (strict)" method="Map XY To Coords"(reference=w495, "XY"=w496) -> ("Coords"=w493:T11)  [unwired: 5 in, 6 out]
                        n159 = Unbundle(w493) -> ("Horizontal"=w501:i32, "Vertical"=w500:i32)
                        n160 = dll-call lib="User32.dll" fn="SetCursorPos"(w501, w500) -> ()  [unwired: 6 in, 2 out]
                      }
                    }
                    n161 = Current VI's Path() -> (path=w471:path)
                    n162 = Strip Path(path=w471) -> (stripped path=w470:path)  [unwired: 1 out]
                    n163 = Build Path(base path=w470, name or relative path="Sounds\\successful_hit.wav") -> (appended path=w472:path)
                    n164 = call <vilib>:"Play Sound File.vi"("path"=w472) -> ()  [unwired: 9 in, 2 out]
                  }
                  frame #1 {
                    w510 = u32 3381759
                    n165 = Subtract(x=w503, y=u32 2) -> (x-y=w507:u32)
                    n166 = To Long Integer(number=w507) -> (32bit integer=w506:i32)
                    n167 = Absolute Value(x=w506) -> (abs(x)=w504:i32)
                    n168 = Add(x=w504, y=u32 1) -> (x+y=w508:u32)
                    n169 = property on="Property Node" class="XYGraph (strict)"(reference=w502, "Active Plot"=w504, "Plot.Fill To"=w508, "Plot.Fill/Pt. Color"=w510, "Plot.Plot Color"=w510) -> ()  [unwired: 1 in, 2 out]
                  }
                  frame #2 {
                    w514 = u32 3223857
                    n170 = property on="Property Node" class="XYGraph (strict)"(reference=w511, "Active Plot"=w513, "Plot.Fill To"=w512, "Plot.Fill/Pt. Color"=w514, "Plot.Plot Color"=w514) -> ()  [unwired: 1 in, 2 out]
                  }
                }
                n171 = call "Active_Target.vi"("Session"=w416, "XYGraph Refnum"=w425) -> ("y0"=w420:dbl, "x0"=w421:dbl)  [unwired: 6 in, 2 out]
                n172 = Add(x=1, y=w418) -> (x+y=w438:i32)
                n173 = Equal?(x=w418, y=0) -> (x = y?=w414:bool)
                n174 = Equal?(x=w416, y=1) -> (x = y?=w413:bool)
                n175 = And(x=w414, y=w413) -> (x .and. y?=w412:bool)
                n176 = Build Array(w421, w420) -> (w419:dbl[])
                n177 = case shown="True" w412 {
                  tunnel: w411 -> [w443 w446]
                  tunnel: [w443 w444] -> w410
                  frame False {
                  }
                  frame True {
                    n178 = Subtract(x=w446, y=1) -> (x-y=w444:i32)
                  }
                }
                n179 = call "InActive_Target.vi"("Session"=w416, "XYGraph Refnum"=w425) -> ("y0"=w423:dbl, "x0"=w424:dbl, "Radius"=w408:dbl)  [unwired: 5 in, 1 out]
                n180 = Build Array(w435, w410) -> (w437:u32[])
                n181 = Build Array(w408, w409) -> (w426:dbl[])
                n182 = Build Array(w424, w423) -> (w422:dbl[])
                n183 = stacked-sequence {
                  tunnel: w437 -> [_ w453 _ _ _]
                  tunnel: w436 -> [w448 w451 w456 w459 w462]
                  tunnel: w426 -> [_ _ w455 _ _]
                  tunnel: w422 -> [_ _ _ w457 _]
                  tunnel: w419 -> [_ _ _ _ w460]
                  tunnel: w406 -> [w449 _ _ _ _]
                  tunnel: [dbl[][] [] _ _ _ _] -> w405
                  frame #0 {
                    n184 = call-poly <vilib>:"Write To Spreadsheet File.vi"("append to file? (new file:F)"=TRUE, "2D data"=w449, "file path (dialog if empty)"=w448) -> ()  [unwired: 5 in, 1 out]
                  }
                  frame #1 {
                    n185 = call-poly <vilib>:"Write To Spreadsheet File.vi"("append to file? (new file:F)"=TRUE, "1D data"=w453, "file path (dialog if empty)"=w451) -> ()  [unwired: 5 in, 1 out]
                  }
                  frame #2 {
                    n186 = call-poly <vilib>:"Write To Spreadsheet File.vi"("append to file? (new file:F)"=TRUE, "1D data"=w455, "file path (dialog if empty)"=w456) -> ()  [unwired: 5 in, 1 out]
                  }
                  frame #3 {
                    n187 = call-poly <vilib>:"Write To Spreadsheet File.vi"("append to file? (new file:F)"=TRUE, "1D data"=w457, "file path (dialog if empty)"=w459) -> ()  [unwired: 5 in, 1 out]
                  }
                  frame #4 {
                    n188 = call-poly <vilib>:"Write To Spreadsheet File.vi"("append to file? (new file:F)"=TRUE, "1D data"=w460, "file path (dialog if empty)"=w462) -> ()  [unwired: 5 in, 1 out]
                  }
                }
                n189 = Multiply(x=w430, y=0) -> (x*y=w428:i32)
                n190 = Multiply(x=w409, y=0) -> (x*y=w427:i32)
                n191 = Multiply(x=w411, y=0) -> (x*y=w432:i32)
              }
            }
          }
        }
        n192 = case shown="True" w162 {
          tunnel: w164 -> [_ w267]
          tunnel: w183 -> [_ _]
          tunnel: w182 -> [_ _]
          tunnel: w205 -> [_ w272]
          tunnel: w202 -> [w265 w271]
          tunnel: [w265 w270] -> w204
          tunnel: w186 -> [_ w269]
          tunnel: w185 -> [_ w268]
          tunnel: w131 -> [w264 _]
          tunnel: [w264 w266] -> w130
          frame False {
          }
          frame True {
            n193 = case shown="True" w272 {
              tunnel: w271 -> [w280 w290]
              tunnel: [w280 w288] -> w270
              tunnel: w269 -> [w279 w284]
              tunnel: w268 -> [w278 w283]
              tunnel: w267 -> [w274 _]
              tunnel: [w273 w281] -> w266
              frame False {
                n194 = Bundle("x0"=w279, "y0"=w278) -> (w277:cluster{"x0":dbl, "y0":dbl})  [unwired: 1 in]
                n195 = invoke on="Invoke Node" class="XYGraph (strict)" method="Map XY To Coords"(reference=w274, "XY"=w277) -> ("Coords"=w273:T11)  [unwired: 5 in, 6 out]
                n196 = Unbundle(w273) -> ("Horizontal"=w276:i32, "Vertical"=w275:i32)
                n197 = dll-call lib="User32.dll" fn="SetCursorPos"(w276, w275) -> ()  [unwired: 6 in, 2 out]
              }
              frame True {
                n198 = Tick Count (ms)() -> (millisecond timer value=→"initial time":u32)
                n199 = Bundle("x0"=w284, "y0"=w283) -> (w287:cluster{"x0":dbl, "y0":dbl})  [unwired: 1 in]
                n200 = invoke on="1D Experiment" class="XYGraph (strict)" method="Map XY To Coords"("XY"=w287) -> ("Coords"=w281:T11)  [unwired: 6 in, 6 out]
                n201 = Unbundle(w281) -> ("Horizontal"=w286:i32, "Vertical"=w285:i32)
                n202 = dll-call lib="User32.dll" fn="SetCursorPos"(w286, w285) -> ()  [unwired: 6 in, 2 out]
                n203 = Add(x=1, y=w290) -> (x+y=w288:i32)
              }
            }
          }
        }
        n204 = node-c288() -> ()  [unwired: 1 in, 1 out]
      }
      n205 = Open/Create/Replace File(file path (use dialog)=w108, operation (0:open)=T1."create") -> (refnum out=w110:refnum<file>)  [unwired: 4 in, 2 out]
      n206 = Open/Create/Replace File(file path (use dialog)=w89, operation (0:open)=T1."create") -> (refnum out=w93:refnum<file>)  [unwired: 4 in, 2 out]
      n207 = Open/Create/Replace File(file path (use dialog)=w88, operation (0:open)=T1."create") -> (refnum out=w91:refnum<file>)  [unwired: 4 in, 2 out]
      n208 = Open/Create/Replace File(file path (use dialog)=w111, operation (0:open)=T1."create") -> (refnum out=w113:refnum<file>)  [unwired: 4 in, 2 out]
      n209 = Open/Create/Replace File(file path (use dialog)=w103, operation (0:open)=T1."create") -> (refnum out=w105:refnum<file>)  [unwired: 4 in, 2 out]
      n210 = Close File(refnum=w110) -> ()  [unwired: 1 in, 2 out]
      n211 = Close File(refnum=w93) -> ()  [unwired: 1 in, 2 out]
      n212 = Close File(refnum=w91) -> ()  [unwired: 1 in, 2 out]
      n213 = Close File(refnum=w113) -> ()  [unwired: 1 in, 2 out]
      n214 = Close File(refnum=w105) -> ()  [unwired: 1 in, 2 out]
      n215 = node-c288(w101) -> ()  [unwired: 1 out]
    }
  }
  n216 = call-poly <vilib>:"Close Input Device.vi"("error in (no error)"=w4, "device ID"=w39) -> ()  [unwired: 9 out]
  n217 = property class="VI"(reference=w20, error in=w19, "Front Panel Window:Open"=TRUE) -> (reference out=w22:refnum<vi>, error out=w21:errorcluster)
  n218 = Close Reference(reference=w22, error in (no error)=w21) -> ()  [unwired: 1 out]
